vi "Get Settings Name.vi"(8 "error in (no error)":errorcluster {"code" format="Error %.0f"}, 11 "Parser Settings In":refnum<class "Parser Settings.lvclass">) -> (0 "error out":errorcluster {"code" format="Error %.0f"}, 2 "Name":string, 3 "Parser Settings Out":refnum<class "Parser Settings.lvclass">)   [LabVIEW 2023, in "VIDoc Parsing.lvlib" / "Parser Settings.lvclass"]
uses:
  Parser Settings.lvclass
  Parser Settings.lvclass/Parser Settings.ctl
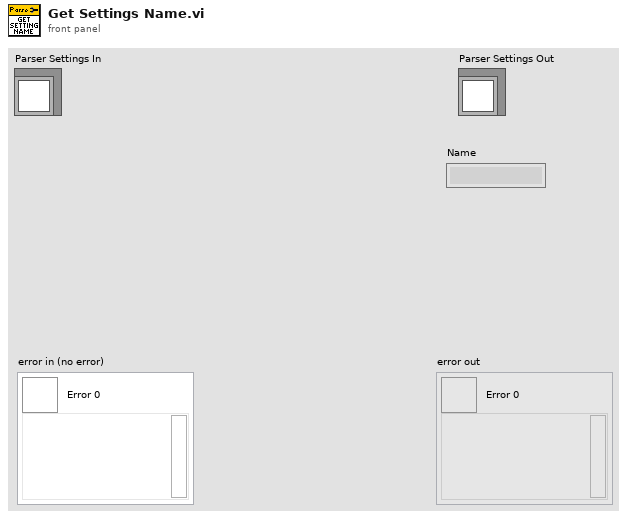
[diagram p1: front panel]
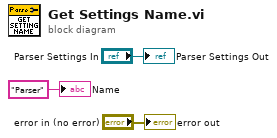
[diagram p0: block diagram]
diagram:
  "error out" <- "error in (no error)"
  "Parser Settings Out" <- "Parser Settings In"
  "Name" <- "Parser" ("Name")
